vi "CRYWindow WAIT CLOSE.vi"(10 "vi reference":refnum<vi>) -> ()   [LabVIEW 2013]
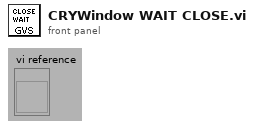
[diagram p1: front panel]
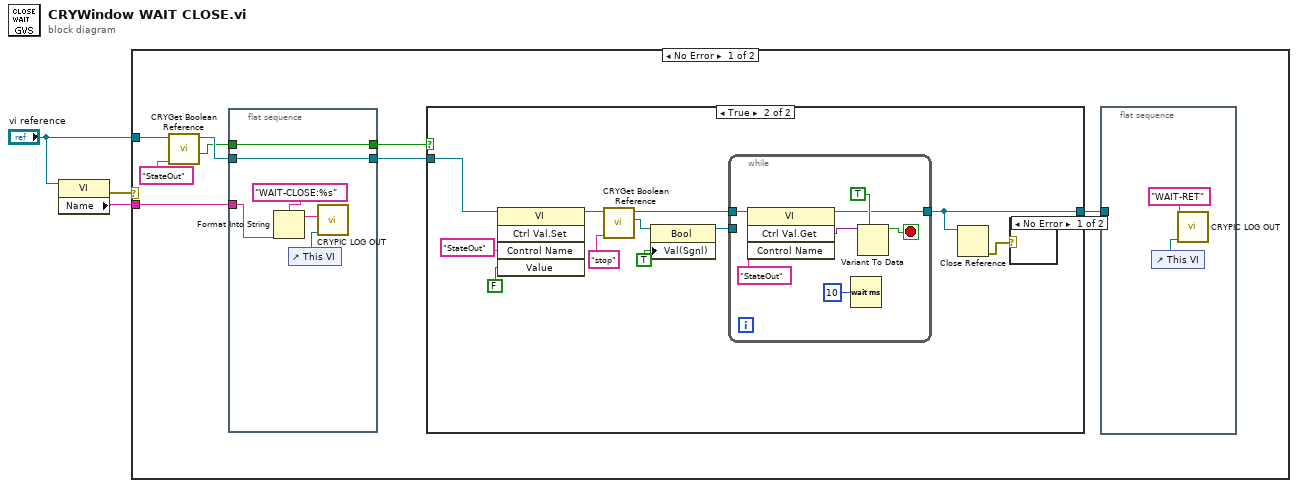
[diagram p0: block diagram]
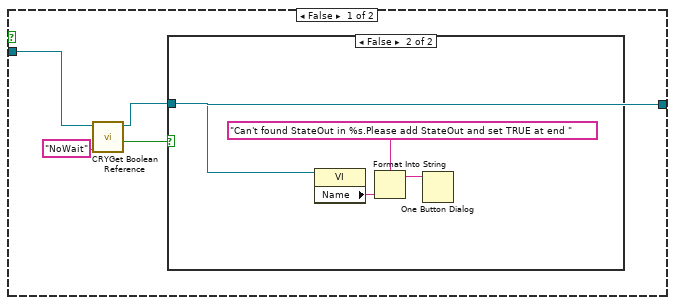
[diagram p2: hidden frame]
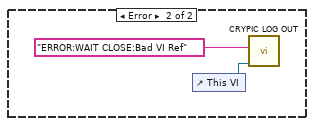
[diagram p5: hidden frame]
diagram:
  n1 = property class="VI"(reference="vi reference") -> (error out=w3:errorcluster, "Name"=w1:string)  [unwired: 1 in, 1 out]
  n2 = case shown="No Error" w3 {
    tunnel: "vi reference" -> [w5 _]
    tunnel: w1 -> [w4 _]
    frame No Error {
      n3 = call "CRYGet Boolean Reference.vi"("Label Name"="StateOut", "VI Refnum"=w5) -> ("Exist?"=w7:bool, "VI Refnum Out"=w8:refnum<vi>)  [unwired: 7 in, 1 out]
      n4 = flat-sequence {
        tunnel: [w43] -> w11
        tunnel: w8 -> [w43]
        tunnel: [w45] -> w6
        tunnel: w7 -> [w45]
        tunnel: w4 -> [w41]
        frame #0 {
          n5 = Format Into String(format string="WAIT-CLOSE:%s", w41) -> (resulting string=w42:string)  [unwired: 2 in, 1 out]
          n6 = control-ref of="This VI"() -> (w40:refnum<vi>)
          n7 = call "CRYPIC LOG OUT.vi"("pVIRef"=w40, "sData"=w42) -> ()  [unwired: 10 in]
        }
      }
      n8 = case shown="True" w6 {
        tunnel: w11 -> [w14 w23]
        tunnel: [w13 w21] -> w10
        frame False {
          n9 = call "CRYGet Boolean Reference.vi"("Label Name"="NoWait", "VI Refnum"=w14) -> ("Exist?"=w12:bool, "VI Refnum Out"=w13:refnum<vi>)  [unwired: 7 in, 1 out]
          n10 = case shown="False" w12 {
            tunnel: w13 -> [_ w16]
            frame True {
            }
            frame False {
              n11 = property class="VI"(reference=w16) -> ("Name"=w18:string)  [unwired: 1 in, 2 out]
              n12 = Format Into String(format string="Can't found StateOut in %s.Please add StateOut and set TRUE at end " ("message"), w18) -> (resulting string=w17:string)  [unwired: 2 in, 1 out]
              n13 = One Button Dialog(message=w17) -> ()  [unwired: 1 in, 1 out]
            }
          }
        }
        frame True {
          n14 = invoke class="VI" method="Ctrl Val.Set"(reference=w23, "Control Name"="StateOut", "Value"=FALSE) -> (reference out=w25:refnum<vi>)  [unwired: 2 in, 4 out]
          n15 = call "CRYGet Boolean Reference.vi"("Label Name"="stop", "VI Refnum"=w25) -> ("Boolean Ref"=w28:refnum<vi>, "VI Refnum Out"=w24:refnum<vi>)  [unwired: 7 in, 1 out]
          n16 = property class="Bool"(reference=w28, "Val(Sgnl)"=TRUE) -> (reference out=w22:refnum<vi>)  [unwired: 1 in, 1 out]
          n17 = while {
            tunnel: w24 -> [w36]
            tunnel: [w32] -> w21
            tunnel: w22 -> [_]
            stop <- w33 stop-if-true
            n18 = invoke class="VI" method="Ctrl Val.Get"(reference=w36, "Control Name"="StateOut") -> (reference out=w32:refnum<vi>, "Get Control Value Variant"=w35:variant)  [unwired: 2 in, 2 out]
            n19 = Wait (ms)(milliseconds to wait=u32 10) -> ()  [unwired: 1 out]
            n20 = Variant To Data(type=TRUE, Variant=w35) -> (data=w33:bool)  [unwired: 1 in, 1 out]
          }
          n21 = Close Reference(reference=w21) -> (error out=w20:errorcluster)  [unwired: 1 in]
          n22 = case shown="No Error" w20 {
            frame No Error {
            }
            frame Error {
            }
          }
        }
      }
      n23 = flat-sequence {
        tunnel: w10 -> [_]
        frame #0 {
          n24 = control-ref of="This VI"() -> (w38:refnum<vi>)
          n25 = call "CRYPIC LOG OUT.vi"("pVIRef"=w38, "sData"="WAIT-RET") -> ()  [unwired: 10 in]
        }
      }
    }
    frame Error {
      n26 = control-ref of="This VI"() -> (w46:refnum<vi>)
      n27 = call "CRYPIC LOG OUT.vi"("pVIRef"=w46, "sData"="ERROR:WAIT CLOSE:Bad VI Ref" ("format string")) -> ()  [unwired: 10 in]
    }
  }
